vi "7_1_2.vi"() -> ()   [LabVIEW 2021, in "2022.lvlib"]
uses:
  2022.lvlib
  <vilib>/National Instruments/Tree Map/Tree Map Data.ctl
  <vilib>/National Instruments/Tree Map/Tree Map.lvlib
panel:
  out "min value":i32
  out "Array 4":i32[](array[numeric])
  out "Array 3":string[](array[string])
  out "x = y? 2":bool
  out "x-y":i32
  out "sum":i32
  out "Array 2":i32[](array[numeric])
  out "Array":string[](array[string])
  out "x = y?":bool
  out "Tree Control Items":T1(array[cluster])
  out "size(s)":i32
  out "Numeric":i32
  out "Tree Map Out":T2
  in  "Tree Control":string(tree)
  out "substring":string
  out "subarray":string[](array[string])
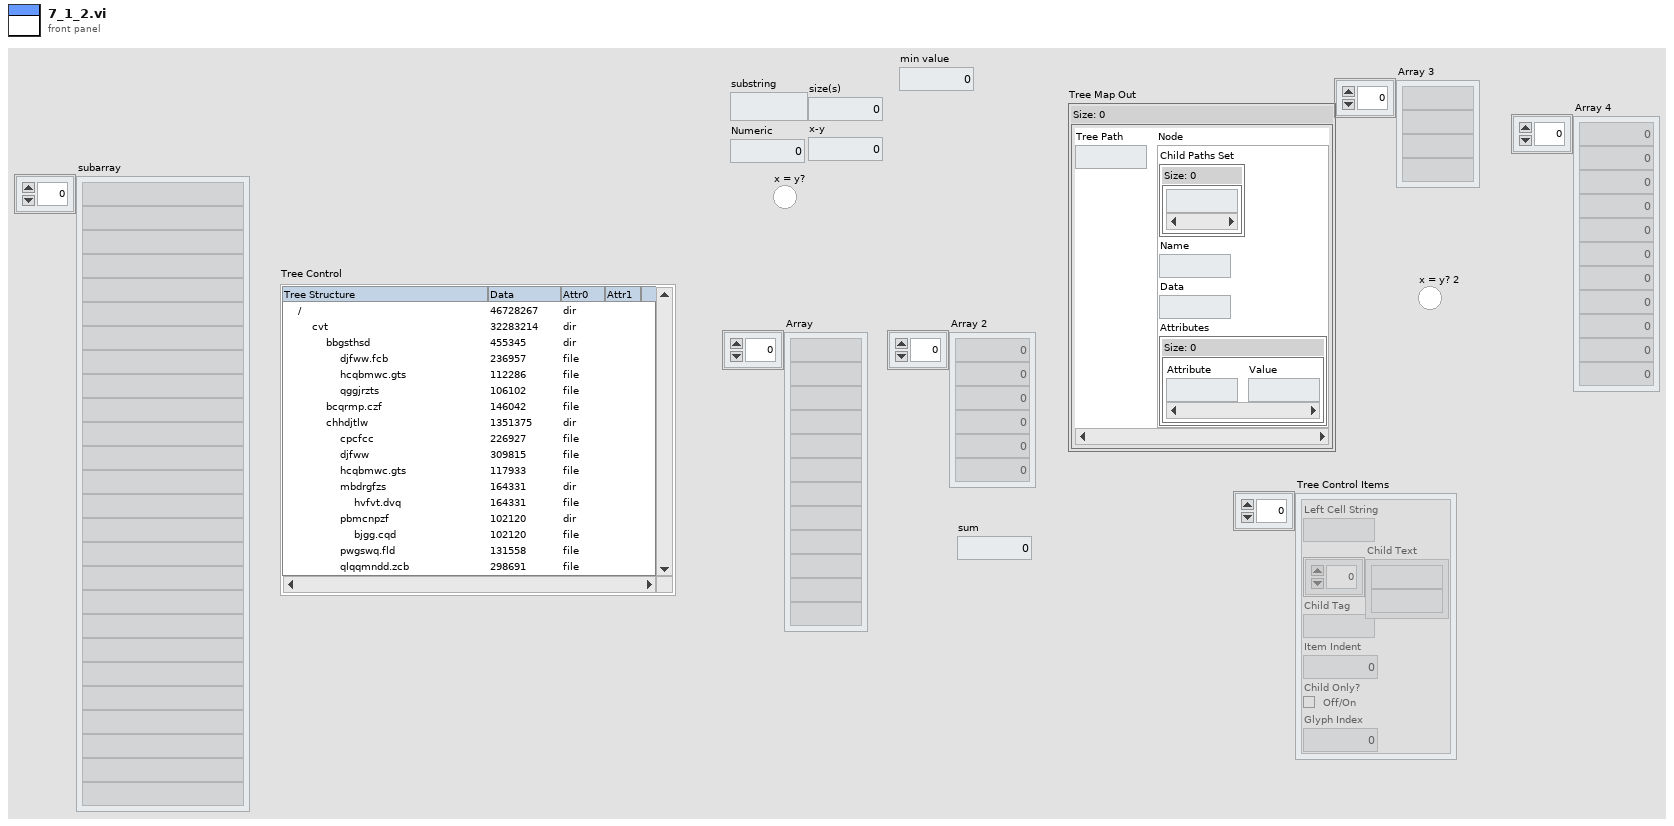
[diagram p1: front panel]
types:
  T1 = cluster{"Left Cell String":string, "Child Text":string[], "Child Tag":string, "Item Indent":i32, "Child Only?":bool, "Glyph Index":i32}[]
  T2 = typedef "Tree Map.lvlib/Tree Map Data.ctl" = map{string, cluster{"Child Paths Set":set{string}, "Name":string, "Data":string, "Attributes":map{string, string}}}
  T3 = cluster{"Child Paths Set":set{string}, "Name":string, "Data":string, "Attributes":map{string, string}}
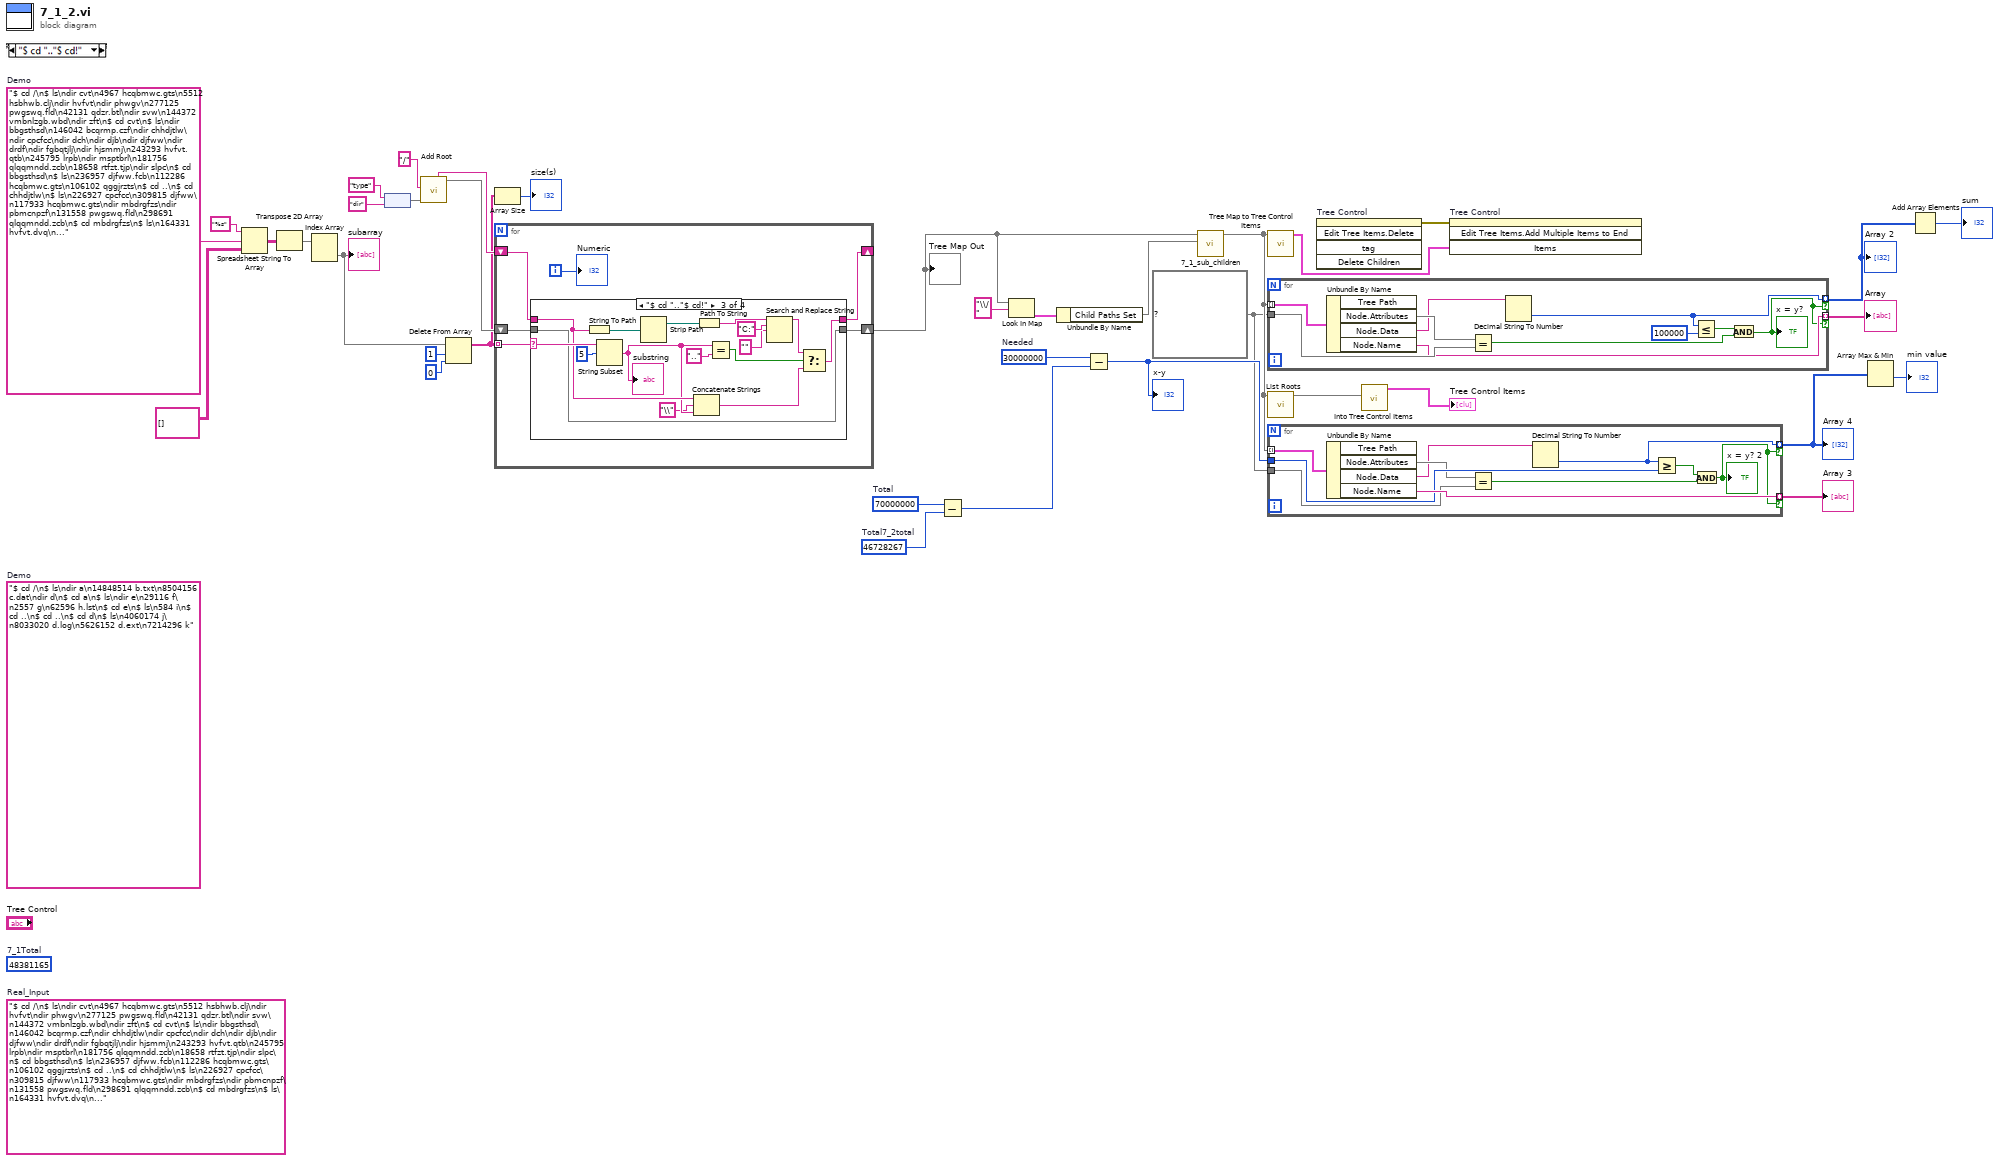
[diagram p0: block diagram]
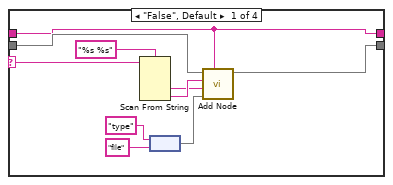
[diagram p2: hidden frame]
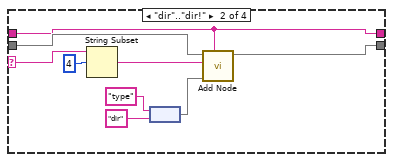
[diagram p3: hidden frame]
diagram:
  (unwired) 48381165  # 7_1Total
  w9 = 70000000  # Total
  w11 = 30000000  # Needed
  w1 = 46728267  # Total7_2total
  w2 = "$ cd /\n$ ls\ndir cvt\n4967 hcqbmwc.gts\n5512 hsbhwb.clj\ndir hvfvt\ndir phwgv\n277125 pwgswq.fld\n42131 qdzr.btl\ndir svw\n144372 vmbnlzgb.wbd\ndir zft\n$ cd cvt\n$ ls\ndir bbgsthsd\n146042 bcqrmp.czf\ndir chhdjtlw\ndir cpcfcc\ndir dch\ndir djb\ndir djfww\ndir drdf\ndir fgbqtjlj\ndir hjsmmj\n243293 hvfvt.qtb\n245795 lrpb\ndir msptbrl\n181756 qlqqmndd.zcb\n18658 rtfzt.tjp\ndir slpc\n$ cd bbgsthsd\n$ ls\n236957 djfww.fcb\n112286 hcqbmwc.gts\n106102 qggjrzts\n$ cd ..\n$ cd chhdjtlw\n$ ls\n226927 cpcfcc\n309815 djfww\n117933 hcqbmwc.gts\ndir mbdrgfzs\ndir pbmcnpzf\n131558 pwgswq.fld\n298691 qlqqmndd.zcb\n$ cd mbdrgfzs\n$ ls\n164331 hvfvt.dvq\n$ cd ..\n$ cd pbmcnpzf\n$ ls\n102120 bjgg.cqd\n$ cd ..\n$ cd ..\n$ cd cpcfcc\n$ ls\n15756 ddc\ndir dqc\ndir glm\ndir jbszm\n200345 pwgswq.fld\n145508 qlqqmndd.zcb\ndir vcptbw\ndir zrtm\n$ cd dqc\n$ ls\ndir cpcfcc\n92063 mzp\ndir qmhnvmh\ndir snqqcjlw\n8423 zdjwr.blc\n$ cd cpcfcc\n$ ls\ndir hvfvt\n$ cd hvfvt\n$ ls\n289372 pwgswq.fld\n307397 qlqqmndd.zcb\n$ cd ..\n$ cd ..\n$ cd qmhnvmh\n$ ls\n274778 jczjwdl.smd\n194322 ngrrfm\n$ cd ..\n$ cd snqqcjlw\n$ ls\n182851 nprvrgd.tbb\n$ cd ..\n$ cd ..\n$ cd glm\n$ ls\n188702 hpq.hgm\n$ cd ..\n$ cd jbszm\n$ ls\n187645 pwgswq.fld\n$ cd ..\n$ cd vcptbw\n$ ls\ndir mgqd\n$ cd mgqd\n$ ls\n157695 rhldvntj.jzm\n268696 rjnngctw\n$ cd ..\n$ cd ..\n$ cd zrtm\n$ ls\n218820 bcqrmp.czf\n172319 czpsl.dnf\n180114 hcqbmwc.gts\n165216 hvfvt.nnw\ndir zft\n$ cd zft\n$ ls\n161245 dtqjg.czv\n249888 hpq.hgm\n192037 zft\n$ cd ..\n$ cd ..\n$ cd ..\n$ cd dch\n$ ls\ndir djfww\ndir fzqgwwnf\ndir hqvmq\ndir mmcrzqc\n42136 qlqqmndd.zcb\ndir vdtlh\ndir wfltm\n271200 zrtm\n$ cd djfww\n$ ls\n37427 dct\n204401 hcqbmwc.gts\n283140 jmq\ndir lbrhbc\n154148 pncb.bmp\n53366 vzt.cnn\n$ cd lbrhbc\n$ ls\ndir djfww\n153648 djfww.pps\n308911 mvtjzp.btg\n219150 ncmc\n253604 wqft.ggb\n293759 zft\n$ cd djfww\n$ ls\n24794 hcqbmwc.gts\n$ cd ..\n$ cd ..\n$ cd ..\n$ cd fzqgwwnf\n$ ls\n233720 scdd.pwr\n$ cd ..\n$ cd hqvmq\n$ ls\ndir cdld\ndir cpcfcc\ndir djfww\n85564 hpq.hgm\ndir qnc\n81509 wtnl.crs\n$ cd cdld\n$ ls\n293421 llpltsgn.tqb\n$ cd ..\n$ cd cpcfcc\n$ ls\n230813 cglljgv\n178203 qlqqmndd.zcb\n186410 zrtm.tbt\n$ cd ..\n$ cd djfww\n$ ls\n201830 zrtm\n$ cd ..\n$ cd qnc\n$ ls\n305356 bdf.jrh\ndir zrtm\n$ cd zrtm\n$ ls\ndir bdhdrr\n$ cd bdhdrr\n$ ls\ndir nffdrnb\n$ cd nffdrnb\n$ ls\n301601 nbrjz\n$ cd ..\n$ cd ..\n$ cd ..\n$ cd ..\n$ cd ..\n$ cd mmcrzqc\n$ ls\ndir cpcfcc\n264271 hpq.hgm\n208744 tzsjrf.zdc\n274096 zft\n$ cd cpcfcc\n$ ls\n226054 cpcfcc\n$ cd ..\n$ cd ..\n$ cd vdtlh\n$ ls\n84229 bzlg.crn\n58668 cpcfcc.zqw\n141409 hpq.hgm\ndir mdgst\n37090 pstsh.qwv\n40357 qlqqmndd.zcb\ndir smr\ndir sqbgcsgh\ndir trp\n$ cd mdgst\n$ ls\n151033 fsmvbpsl.nqr\n$ cd ..\n$ cd smr\n$ ls\n140764 cpcfcc.dpg\n$ cd ..\n$ cd sqbgcsgh\n$ ls\ndir djfww\n263783 dvm\n105219 hpq.hgm\n29647 hwcgv.gvg\n162537 lwjhgh.wmt\n235511 nlw\ndir zwddrdfz\n$ cd djfww\n$ ls\n260084 vcgpvpd\n$ cd ..\n$ cd zwddrdfz\n$ ls\n225632 bhrzzw\n269756 cqq.vrz\n$ cd ..\n$ cd ..\n$ cd trp\n$ ls\n233192 vqwngcs\n$ cd ..\n$ cd ..\n$ cd wfltm\n$ ls\n140990 djfww\n$ cd ..\n$ cd ..\n$ cd djb\n$ ls\n213191 cjwrs.prd\ndir dhvpqt\ndir gtgftm\ndir hvfvt\n208325 jwhp\n301446 qlqqmndd.zcb\ndir qnlbgvf\ndir tps\ndir zft\ndir zrtm\ndir zwnlm\n$ cd dhvpqt\n$ ls\ndir sbcj\n$ cd sbcj\n$ ls\n20611 ggt\n$ cd ..\n$ cd ..\n$ cd gtgftm\n$ ls\n179526 qcqbtmvq\n$ cd ..\n$ cd hvfvt\n$ ls\ndir djstcnrt\ndir hggpvn\ndir hvfvt\n63889 hvfvt.tjm\n265836 qlqqmndd.zcb\n105663 zft\n223582 zft.llg\n26037 zzwwg.lqh\n$ cd djstcnrt\n$ ls\n201498 hcqbmwc.gts\n139156 hpq.hgm\n277342 pshgz.rtp\ndir rjb\n257294 rqrb.lhh\ndir tqnbfnt\n313308 zft.dvc\n$ cd rjb\n$ ls\n268438 hpq.hgm\ndir hvfvt\ndir hvwpb\n161024 mzbcgqc.nvw\n137875 pwgswq.fld\n260008 pzzcww\n283261 wnvlrg.tmn\n$ cd hvfvt\n$ ls\ndir dvwqqt\n163397 hcqbmwc.gts\n265154 pwgswq.fld\ndir trsh\ndir vnf\n$ cd dvwqqt\n$ ls\n315187 hcqbmwc.gts\n$ cd ..\n$ cd trsh\n$ ls\ndir ssrdpg\n$ cd ssrdpg\n$ ls\ndir vjdc\n$ cd vjdc\n$ ls\ndir srvdrhdq\n$ cd srvdrhdq\n$ ls\n74145 djfww\n$ cd ..\n$ cd ..\n$ cd ..\n$ cd ..\n$ cd vnf\n$ ls\ndir djfww\n$ cd djfww\n$ ls\n184018 pwgswq.fld\n$ cd ..\n$ cd ..\n$ cd ..\n$ cd hvwpb\n$ ls\ndir jwpjrcvs\n$ cd jwpjrcvs\n$ ls\ndir cpcfcc\n$ cd cpcfcc\n$ ls\n52191 sdlv\n$ cd ..\n$ cd ..\n$ cd ..\n$ cd ..\n$ cd tqnbfnt\n$ ls\ndir djfww\n206341 fmpb.lnp\ndir fpsjg\n4589 hcqbmwc.gts\ndir hvfvt\n8796 hvfvt.hdz\n238364 tgcdpjc.fjm\ndir zrtm\n40577 zrtm.fsr\n$ cd djfww\n$ ls\n217182 djfww.rbf\n$ cd ..\n$ cd fpsjg\n$ ls\n52456 djfww\n$ cd ..\n$ cd hvfvt\n$ ls\ndir rqhzvb\n275026 szwgzm.qjd\ndir zbmtstj\n$ cd rqhzvb\n$ ls\n8395 gcmzsd.jzf\n$ cd ..\n$ cd zbmtstj\n$ ls\n39691 qlqqmndd.zcb\ndir qqcdss\n180676 rwl.zwr\n$ cd qqcdss\n$ ls\n106297 zrtm.nsl\n$ cd ..\n$ cd ..\n$ cd ..\n$ cd zrtm\n$ ls\n153478 ldhvt\n$ cd ..\n$ cd ..\n$ cd ..\n$ cd hggpvn\n$ ls\n19109 cpcfcc.fbh\n249168 fnqjc\n207420 qgzsh.pfs\n135472 qlqqmndd.zcb\n$ cd ..\n$ cd hvfvt\n$ ls\ndir djfww\n213659 hcqbmwc.gts\ndir jzdwq\n204021 nvbgf\n185328 qlqqmndd.zcb\ndir zrtm\n$ cd djfww\n$ ls\n180713 rwmm.gjt\n$ cd ..\n$ cd jzdwq\n$ ls\n57424 djfww.qtm\n104960 slq.bfp\n174906 svc\n$ cd ..\n$ cd zrtm\n$ ls\ndir mrtvhht\n$ cd mrtvhht\n$ ls\n188512 djfww.fvm\n$ cd ..\n$ cd ..\n$ cd ..\n$ cd ..\n$ cd qnlbgvf\n$ ls\ndir fjrhtssv\n46767 jhbnml.lpq\n$ cd fjrhtssv\n$ ls\n198664 fgcc\n245142 tsc.rsd\n$ cd ..\n$ cd ..\n$ cd tps\n$ ls\ndir fmlwghjv\n146731 gwch.ttr\ndir jjzmdd\ndir rtltrng\n191609 wff.mqt\n$ cd fmlwghjv\n$ ls\n189227 zrtm.vgg\n$ cd ..\n$ cd jjzmdd\n$ ls\ndir hvfvt\n178057 mpdfrrm\n49493 pwgswq.fld\n220129 sqgfb.flm\n231012 zrmsnmr\n$ cd hvfvt\n$ ls\ndir lbndbhc\n12602 mnclbss\n746 ppw\n$ cd lbndbhc\n$ ls\n49601 cdqvs.gwc\n158670 wvjpchjg\n$ cd ..\n$ cd ..\n$ cd ..\n$ cd rtltrng\n$ ls\ndir cpgh\n115613 hvfvt\n59441 zfs\n$ cd cpgh\n$ ls\ndir djfww\n$ cd djfww\n$ ls\ndir tgt\n$ cd tgt\n$ ls\ndir vqwvqss\n$ cd vqwvqss\n$ ls\ndir bsdrhz\n$ cd bsdrhz\n$ ls\ndir pld\n$ cd pld\n$ ls\n8543 mfs.gsb\n$ cd ..\n$ cd ..\n$ cd ..\n$ cd ..\n$ cd ..\n$ cd ..\n$ cd ..\n$ cd ..\n$ cd zft\n$ ls\ndir fhjgg\n$ cd fhjgg\n$ ls\n114494 pwgswq.fld\n$ cd ..\n$ cd ..\n$ cd zrtm\n$ ls\n201142 tlhr.rtd\n298232 wlcztszv\n$ cd ..\n$ cd zwnlm\n$ ls\n240023 hcqbmwc.gts\n159126 hpq.hgm\n22101 hvfvt.bfw\ndir ltzl\ndir mtfr\ndir sbw\ndir sqscdjlj\ndir ssf\n$ cd ltzl\n$ ls\n260692 hpq.hgm\n204540 hvfvt\n$ cd ..\n$ cd mtfr\n$ ls\n15391 pwgswq.fld\n$ cd ..\n$ cd sbw\n$ ls\n293226 hcqbmwc.gts\n267478 htllcq\n176349 nlbhcf.vpn\n286577 zft.gds\n$ cd ..\n$ cd sqscdjlj\n$ ls\n128776 gnh\ndir qbdpvcbt\n284505 qlsn.vdq\n$ cd qbdpvcbt\n$ ls\n280709 crv.hgm\n$ cd ..\n$ cd ..\n$ cd ssf\n$ ls\n13328 djfww.pjn\n19971 hvfvt\ndir zft\n$ cd zft\n$ ls\n97761 dnmnz\n$ cd ..\n$ cd ..\n$ cd ..\n$ cd ..\n$ cd djfww\n$ ls\n109590 bwfnnf.wpd\n297297 cmht.ljg\n280726 hvfvt\n$ cd ..\n$ cd drdf\n$ ls\n56764 pwgswq.fld\n300547 wqqm\n210698 zrtm.jvq\n$ cd ..\n$ cd fgbqtjlj\n$ ls\n22217 vrmgsz.ctg\n$ cd ..\n$ cd hjsmmj\n$ ls\n232911 bcqrmp.czf\n164656 hcqbmwc.gts\ndir jql\ndir ntd\ndir prgm\ndir psfvhh\ndir zft\n$ cd jql\n$ ls\n212767 zhnhn.lzm\ndir zrtm\n$ cd zrtm\n$ ls\n35950 bcqrmp.czf\n$ cd ..\n$ cd ..\n$ cd ntd\n$ ls\ndir vml\n$ cd vml\n$ ls\n60833 bcqrmp.czf\n$ cd ..\n$ cd ..\n$ cd prgm\n$ ls\n316166 pwgswq.fld\n$ cd ..\n$ cd psfvhh\n$ ls\n152195 pwgswq.fld\n92448 qlqqmndd.zcb\n$ cd ..\n$ cd zft\n$ ls\n95808 hpq.hgm\n$ cd ..\n$ cd ..\n$ cd msptbrl\n$ ls\n256069 hpq.hgm\n$ cd ..\n$ cd slpc\n$ ls\ndir djfww\n285380 djfww.gcm\n169898 hcqbmwc.gts\n40914 mnpnhpz\n188062 pwgswq.fld\ndir zrtm\n$ cd djfww\n$ ls\n94935 pwgswq.fld\n70655 qlqqmndd.zcb\n48528 zft.qvh\n$ cd ..\n$ cd zrtm\n$ ls\n160137 hcqbmwc.gts\n$ cd ..\n$ cd ..\n$ cd ..\n$ cd hvfvt\n$ ls\ndir cslthslv\n129407 prwq\ndir vrzfbtt\n$ cd cslthslv\n$ ls\ndir cpcfcc\n158361 hcqbmwc.gts\n$ cd cpcfcc\n$ ls\ndir zpgnczq\n$ cd zpgnczq\n$ ls\n158414 zft\n$ cd ..\n$ cd ..\n$ cd ..\n$ cd vrzfbtt\n$ ls\n185263 nqvvl\n$ cd ..\n$ cd ..\n$ cd phwgv\n$ ls\n253690 bzpcj.fcj\ndir wtbr\n168025 zdsh.tnq\n157840 zsdfqb.zbd\n$ cd wtbr\n$ ls\ndir lvgdb\n$ cd lvgdb\n$ ls\n177751 cpcfcc.dzr\n$ cd ..\n$ cd ..\n$ cd ..\n$ cd svw\n$ ls\ndir cpcfcc\n189430 hpq.hgm\ndir ntzbj\n13384 qlqqmndd.zcb\n10333 wdvqhwgl.trq\n161318 zwzp.jsn\n$ cd cpcfcc\n$ ls\n298999 hcqbmwc.gts\n290883 hpq.hgm\ndir qlnntp\ndir vpshs\n5547 wlrmg.bpc\ndir zft\n$ cd qlnntp\n$ ls\n168562 nqds.tqn\n$ cd ..\n$ cd vpshs\n$ ls\n246400 pwgswq.fld\n$ cd ..\n$ cd zft\n$ ls\n235634 hvfvt.hst\n$ cd ..\n$ cd ..\n$ cd ntzbj\n$ ls\n98777 qlqqmndd.zcb\n$ cd ..\n$ cd ..\n$ cd zft\n$ ls\ndir dhnzm\n299292 hvfvt.pvb\ndir ltfb\ndir mrvsjgsq\ndir ntr\ndir swmvhgd\ndir zrtm\n$ cd dhnzm\n$ ls\n267041 bbsj\n$ cd ..\n$ cd ltfb\n$ ls\n242136 bcqrmp.czf\n314862 dgdz\n203160 hcqbmwc.gts\n80422 hgvz\ndir qftjfqfv\n180815 sstl.wzg\ndir wmhm\ndir zft\ndir zszp\n$ cd qftjfqfv\n$ ls\ndir bmmw\n$ cd bmmw\n$ ls\ndir hvfvt\n318039 hvfvt.whc\n17057 pwgswq.fld\n$ cd hvfvt\n$ ls\n170348 brplf.wgv\n156783 hcqbmwc.gts\n$ cd ..\n$ cd ..\n$ cd ..\n$ cd wmhm\n$ ls\n178474 bcqrmp.czf\ndir cmsgv\ndir dcfvrtj\n225393 htjflrs.tlm\ndir hvfvt\ndir nlrs\n273173 nsmdd.glc\n151259 pwgswq.fld\ndir ztqvwjr\n$ cd cmsgv\n$ ls\ndir flgjbjg\n$ cd flgjbjg\n$ ls\n13971 cpcfcc\n20601 qlqqmndd.zcb\n$ cd ..\n$ cd ..\n$ cd dcfvrtj\n$ ls\n141992 djfww.djn\n118149 hpq.hgm\ndir qrmqslq\n$ cd qrmqslq\n$ ls\n105940 zrtm.vql\n$ cd ..\n$ cd ..\n$ cd hvfvt\n$ ls\n181962 hpq.hgm\n$ cd ..\n$ cd nlrs\n$ ls\n82705 vnfwjf.hhl\n$ cd ..\n$ cd ztqvwjr\n$ ls\n98257 pwgswq.fld\n83864 scv.pbp\n$ cd ..\n$ cd ..\n$ cd zft\n$ ls\n183072 rsbfsl.zsj\n$ cd ..\n$ cd zszp\n$ ls\ndir hvfvt\n$ cd hvfvt\n$ ls\ndir djfww\ndir dqdtgjtg\ndir hvfvt\n$ cd djfww\n$ ls\n117037 rnmbsq.zph\n259243 zrtm.znf\n$ cd ..\n$ cd dqdtgjtg\n$ ls\ndir lrbsvng\n59301 zft\n$ cd lrbsvng\n$ ls\n46301 bcqrmp.czf\n$ cd ..\n$ cd ..\n$ cd hvfvt\n$ ls\n223277 qlqqmndd.zcb\n$ cd ..\n$ cd ..\n$ cd ..\n$ cd ..\n$ cd mrvsjgsq\n$ ls\n160189 cpcfcc\ndir lzqf\n232626 pwgswq.fld\ndir rpmfcg\n$ cd lzqf\n$ ls\n135552 bcqrmp.czf\n48083 qlqqmndd.zcb\ndir rbg\n229086 rdswb.cjz\n204486 spbwfrwf.cmj\n$ cd rbg\n$ ls\ndir sjdwsbqq\n$ cd sjdwsbqq\n$ ls\n270621 rhv.shw\n$ cd ..\n$ cd ..\n$ cd ..\n$ cd rpmfcg\n$ ls\n227216 bld.jtn\ndir zft\n$ cd zft\n$ ls\n43056 vzc\n$ cd ..\n$ cd ..\n$ cd ..\n$ cd ntr\n$ ls\ndir cmtnqb\ndir djfww\n195371 wffvmql.lrv\n$ cd cmtnqb\n$ ls\n135380 pbng.vhq\n$ cd ..\n$ cd djfww\n$ ls\ndir fmvrrrq\ndir mbhrbss\ndir zrtm\n$ cd fmvrrrq\n$ ls\ndir cpcfcc\n79110 djfww\n300581 ftcdj.wcc\n$ cd cpcfcc\n$ ls\n234211 zsgsm\n$ cd ..\n$ cd ..\n$ cd mbhrbss\n$ ls\n149184 djfww.gwh\n185815 rhgw.rmj\n$ cd ..\n$ cd zrtm\n$ ls\ndir zft\n$ cd zft\n$ ls\n310043 bnwvt.fbg\n$ cd ..\n$ cd ..\n$ cd ..\n$ cd ..\n$ cd swmvhgd\n$ ls\n77547 djfww.jwr\n318547 drggg\n300962 pwgswq.fld\n$ cd ..\n$ cd zrtm\n$ ls\n229319 bflnffjj\ndir djfww\n142526 hvfvt\n232722 jprrf\n94024 ndmf.hdr\ndir vhdhn\n$ cd djfww\n$ ls\n30770 bcqrmp.czf\n$ cd ..\n$ cd vhdhn\n$ ls\ndir djfww\n48261 djfww.frg\ndir gqc\n316163 qlqqmndd.zcb\n$ cd djfww\n$ ls\n104095 cvjlthn.cfl\n223454 hgqwzh\n24715 pwgswq.fld\n283499 qlqqmndd.zcb\ndir zft\n224574 zlnwn\n$ cd zft\n$ ls\n100941 pwgswq.fld\n$ cd ..\n$ cd ..\n$ cd gqc\n$ ls\n156273 wpgwrdl"  # Demo
  w5 = map{string, string} {"type"="dir"} ("Attributes")
  (unwired) "$ cd /\n$ ls\ndir cvt\n4967 hcqbmwc.gts\n5512 hsbhwb.clj\ndir hvfvt\ndir phwgv\n277125 pwgswq.fld\n42131 qdzr.btl\ndir svw\n144372 vmbnlzgb.wbd\ndir zft\n$ cd cvt\n$ ls\ndir bbgsthsd\n146042 bcqrmp.czf\ndir chhdjtlw\ndir cpcfcc\ndir dch\ndir djb\ndir djfww\ndir drdf\ndir fgbqtjlj\ndir hjsmmj\n243293 hvfvt.qtb\n245795 lrpb\ndir msptbrl\n181756 qlqqmndd.zcb\n18658 rtfzt.tjp\ndir slpc\n$ cd bbgsthsd\n$ ls\n236957 djfww.fcb\n112286 hcqbmwc.gts\n106102 qggjrzts\n$ cd ..\n$ cd chhdjtlw\n$ ls\n226927 cpcfcc\n309815 djfww\n117933 hcqbmwc.gts\ndir mbdrgfzs\ndir pbmcnpzf\n131558 pwgswq.fld\n298691 qlqqmndd.zcb\n$ cd mbdrgfzs\n$ ls\n164331 hvfvt.dvq\n$ cd ..\n$ cd pbmcnpzf\n$ ls\n102120 bjgg.cqd\n$ cd ..\n$ cd ..\n$ cd cpcfcc\n$ ls\n15756 ddc\ndir dqc\ndir glm\ndir jbszm\n200345 pwgswq.fld\n145508 qlqqmndd.zcb\ndir vcptbw\ndir zrtm\n$ cd dqc\n$ ls\ndir cpcfcc\n92063 mzp\ndir qmhnvmh\ndir snqqcjlw\n8423 zdjwr.blc\n$ cd cpcfcc\n$ ls\ndir hvfvt\n$ cd hvfvt\n$ ls\n289372 pwgswq.fld\n307397 qlqqmndd.zcb\n$ cd ..\n$ cd ..\n$ cd qmhnvmh\n$ ls\n274778 jczjwdl.smd\n194322 ngrrfm\n$ cd ..\n$ cd snqqcjlw\n$ ls\n182851 nprvrgd.tbb\n$ cd ..\n$ cd ..\n$ cd glm\n$ ls\n188702 hpq.hgm\n$ cd ..\n$ cd jbszm\n$ ls\n187645 pwgswq.fld\n$ cd ..\n$ cd vcptbw\n$ ls\ndir mgqd\n$ cd mgqd\n$ ls\n157695 rhldvntj.jzm\n268696 rjnngctw\n$ cd ..\n$ cd ..\n$ cd zrtm\n$ ls\n218820 bcqrmp.czf\n172319 czpsl.dnf\n180114 hcqbmwc.gts\n165216 hvfvt.nnw\ndir zft\n$ cd zft\n$ ls\n161245 dtqjg.czv\n249888 hpq.hgm\n192037 zft\n$ cd ..\n$ cd ..\n$ cd ..\n$ cd dch\n$ ls\ndir djfww\ndir fzqgwwnf\ndir hqvmq\ndir mmcrzqc\n42136 qlqqmndd.zcb\ndir vdtlh\ndir wfltm\n271200 zrtm\n$ cd djfww\n$ ls\n37427 dct\n204401 hcqbmwc.gts\n283140 jmq\ndir lbrhbc\n154148 pncb.bmp\n53366 vzt.cnn\n$ cd lbrhbc\n$ ls\ndir djfww\n153648 djfww.pps\n308911 mvtjzp.btg\n219150 ncmc\n253604 wqft.ggb\n293759 zft\n$ cd djfww\n$ ls\n24794 hcqbmwc.gts\n$ cd ..\n$ cd ..\n$ cd ..\n$ cd fzqgwwnf\n$ ls\n233720 scdd.pwr\n$ cd ..\n$ cd hqvmq\n$ ls\ndir cdld\ndir cpcfcc\ndir djfww\n85564 hpq.hgm\ndir qnc\n81509 wtnl.crs\n$ cd cdld\n$ ls\n293421 llpltsgn.tqb\n$ cd ..\n$ cd cpcfcc\n$ ls\n230813 cglljgv\n178203 qlqqmndd.zcb\n186410 zrtm.tbt\n$ cd ..\n$ cd djfww\n$ ls\n201830 zrtm\n$ cd ..\n$ cd qnc\n$ ls\n305356 bdf.jrh\ndir zrtm\n$ cd zrtm\n$ ls\ndir bdhdrr\n$ cd bdhdrr\n$ ls\ndir nffdrnb\n$ cd nffdrnb\n$ ls\n301601 nbrjz\n$ cd ..\n$ cd ..\n$ cd ..\n$ cd ..\n$ cd ..\n$ cd mmcrzqc\n$ ls\ndir cpcfcc\n264271 hpq.hgm\n208744 tzsjrf.zdc\n274096 zft\n$ cd cpcfcc\n$ ls\n226054 cpcfcc\n$ cd ..\n$ cd ..\n$ cd vdtlh\n$ ls\n84229 bzlg.crn\n58668 cpcfcc.zqw\n141409 hpq.hgm\ndir mdgst\n37090 pstsh.qwv\n40357 qlqqmndd.zcb\ndir smr\ndir sqbgcsgh\ndir trp\n$ cd mdgst\n$ ls\n151033 fsmvbpsl.nqr\n$ cd ..\n$ cd smr\n$ ls\n140764 cpcfcc.dpg\n$ cd ..\n$ cd sqbgcsgh\n$ ls\ndir djfww\n263783 dvm\n105219 hpq.hgm\n29647 hwcgv.gvg\n162537 lwjhgh.wmt\n235511 nlw\ndir zwddrdfz\n$ cd djfww\n$ ls\n260084 vcgpvpd\n$ cd ..\n$ cd zwddrdfz\n$ ls\n225632 bhrzzw\n269756 cqq.vrz\n$ cd ..\n$ cd ..\n$ cd trp\n$ ls\n233192 vqwngcs\n$ cd ..\n$ cd ..\n$ cd wfltm\n$ ls\n140990 djfww\n$ cd ..\n$ cd ..\n$ cd djb\n$ ls\n213191 cjwrs.prd\ndir dhvpqt\ndir gtgftm\ndir hvfvt\n208325 jwhp\n301446 qlqqmndd.zcb\ndir qnlbgvf\ndir tps\ndir zft\ndir zrtm\ndir zwnlm\n$ cd dhvpqt\n$ ls\ndir sbcj\n$ cd sbcj\n$ ls\n20611 ggt\n$ cd ..\n$ cd ..\n$ cd gtgftm\n$ ls\n179526 qcqbtmvq\n$ cd ..\n$ cd hvfvt\n$ ls\ndir djstcnrt\ndir hggpvn\ndir hvfvt\n63889 hvfvt.tjm\n265836 qlqqmndd.zcb\n105663 zft\n223582 zft.llg\n26037 zzwwg.lqh\n$ cd djstcnrt\n$ ls\n201498 hcqbmwc.gts\n139156 hpq.hgm\n277342 pshgz.rtp\ndir rjb\n257294 rqrb.lhh\ndir tqnbfnt\n313308 zft.dvc\n$ cd rjb\n$ ls\n268438 hpq.hgm\ndir hvfvt\ndir hvwpb\n161024 mzbcgqc.nvw\n137875 pwgswq.fld\n260008 pzzcww\n283261 wnvlrg.tmn\n$ cd hvfvt\n$ ls\ndir dvwqqt\n163397 hcqbmwc.gts\n265154 pwgswq.fld\ndir trsh\ndir vnf\n$ cd dvwqqt\n$ ls\n315187 hcqbmwc.gts\n$ cd ..\n$ cd trsh\n$ ls\ndir ssrdpg\n$ cd ssrdpg\n$ ls\ndir vjdc\n$ cd vjdc\n$ ls\ndir srvdrhdq\n$ cd srvdrhdq\n$ ls\n74145 djfww\n$ cd ..\n$ cd ..\n$ cd ..\n$ cd ..\n$ cd vnf\n$ ls\ndir djfww\n$ cd djfww\n$ ls\n184018 pwgswq.fld\n$ cd ..\n$ cd ..\n$ cd ..\n$ cd hvwpb\n$ ls\ndir jwpjrcvs\n$ cd jwpjrcvs\n$ ls\ndir cpcfcc\n$ cd cpcfcc\n$ ls\n52191 sdlv\n$ cd ..\n$ cd ..\n$ cd ..\n$ cd ..\n$ cd tqnbfnt\n$ ls\ndir djfww\n206341 fmpb.lnp\ndir fpsjg\n4589 hcqbmwc.gts\ndir hvfvt\n8796 hvfvt.hdz\n238364 tgcdpjc.fjm\ndir zrtm\n40577 zrtm.fsr\n$ cd djfww\n$ ls\n217182 djfww.rbf\n$ cd ..\n$ cd fpsjg\n$ ls\n52456 djfww\n$ cd ..\n$ cd hvfvt\n$ ls\ndir rqhzvb\n275026 szwgzm.qjd\ndir zbmtstj\n$ cd rqhzvb\n$ ls\n8395 gcmzsd.jzf\n$ cd ..\n$ cd zbmtstj\n$ ls\n39691 qlqqmndd.zcb\ndir qqcdss\n180676 rwl.zwr\n$ cd qqcdss\n$ ls\n106297 zrtm.nsl\n$ cd ..\n$ cd ..\n$ cd ..\n$ cd zrtm\n$ ls\n153478 ldhvt\n$ cd ..\n$ cd ..\n$ cd ..\n$ cd hggpvn\n$ ls\n19109 cpcfcc.fbh\n249168 fnqjc\n207420 qgzsh.pfs\n135472 qlqqmndd.zcb\n$ cd ..\n$ cd hvfvt\n$ ls\ndir djfww\n213659 hcqbmwc.gts\ndir jzdwq\n204021 nvbgf\n185328 qlqqmndd.zcb\ndir zrtm\n$ cd djfww\n$ ls\n180713 rwmm.gjt\n$ cd ..\n$ cd jzdwq\n$ ls\n57424 djfww.qtm\n104960 slq.bfp\n174906 svc\n$ cd ..\n$ cd zrtm\n$ ls\ndir mrtvhht\n$ cd mrtvhht\n$ ls\n188512 djfww.fvm\n$ cd ..\n$ cd ..\n$ cd ..\n$ cd ..\n$ cd qnlbgvf\n$ ls\ndir fjrhtssv\n46767 jhbnml.lpq\n$ cd fjrhtssv\n$ ls\n198664 fgcc\n245142 tsc.rsd\n$ cd ..\n$ cd ..\n$ cd tps\n$ ls\ndir fmlwghjv\n146731 gwch.ttr\ndir jjzmdd\ndir rtltrng\n191609 wff.mqt\n$ cd fmlwghjv\n$ ls\n189227 zrtm.vgg\n$ cd ..\n$ cd jjzmdd\n$ ls\ndir hvfvt\n178057 mpdfrrm\n49493 pwgswq.fld\n220129 sqgfb.flm\n231012 zrmsnmr\n$ cd hvfvt\n$ ls\ndir lbndbhc\n12602 mnclbss\n746 ppw\n$ cd lbndbhc\n$ ls\n49601 cdqvs.gwc\n158670 wvjpchjg\n$ cd ..\n$ cd ..\n$ cd ..\n$ cd rtltrng\n$ ls\ndir cpgh\n115613 hvfvt\n59441 zfs\n$ cd cpgh\n$ ls\ndir djfww\n$ cd djfww\n$ ls\ndir tgt\n$ cd tgt\n$ ls\ndir vqwvqss\n$ cd vqwvqss\n$ ls\ndir bsdrhz\n$ cd bsdrhz\n$ ls\ndir pld\n$ cd pld\n$ ls\n8543 mfs.gsb\n$ cd ..\n$ cd ..\n$ cd ..\n$ cd ..\n$ cd ..\n$ cd ..\n$ cd ..\n$ cd ..\n$ cd zft\n$ ls\ndir fhjgg\n$ cd fhjgg\n$ ls\n114494 pwgswq.fld\n$ cd ..\n$ cd ..\n$ cd zrtm\n$ ls\n201142 tlhr.rtd\n298232 wlcztszv\n$ cd ..\n$ cd zwnlm\n$ ls\n240023 hcqbmwc.gts\n159126 hpq.hgm\n22101 hvfvt.bfw\ndir ltzl\ndir mtfr\ndir sbw\ndir sqscdjlj\ndir ssf\n$ cd ltzl\n$ ls\n260692 hpq.hgm\n204540 hvfvt\n$ cd ..\n$ cd mtfr\n$ ls\n15391 pwgswq.fld\n$ cd ..\n$ cd sbw\n$ ls\n293226 hcqbmwc.gts\n267478 htllcq\n176349 nlbhcf.vpn\n286577 zft.gds\n$ cd ..\n$ cd sqscdjlj\n$ ls\n128776 gnh\ndir qbdpvcbt\n284505 qlsn.vdq\n$ cd qbdpvcbt\n$ ls\n280709 crv.hgm\n$ cd ..\n$ cd ..\n$ cd ssf\n$ ls\n13328 djfww.pjn\n19971 hvfvt\ndir zft\n$ cd zft\n$ ls\n97761 dnmnz\n$ cd ..\n$ cd ..\n$ cd ..\n$ cd ..\n$ cd djfww\n$ ls\n109590 bwfnnf.wpd\n297297 cmht.ljg\n280726 hvfvt\n$ cd ..\n$ cd drdf\n$ ls\n56764 pwgswq.fld\n300547 wqqm\n210698 zrtm.jvq\n$ cd ..\n$ cd fgbqtjlj\n$ ls\n22217 vrmgsz.ctg\n$ cd ..\n$ cd hjsmmj\n$ ls\n232911 bcqrmp.czf\n164656 hcqbmwc.gts\ndir jql\ndir ntd\ndir prgm\ndir psfvhh\ndir zft\n$ cd jql\n$ ls\n212767 zhnhn.lzm\ndir zrtm\n$ cd zrtm\n$ ls\n35950 bcqrmp.czf\n$ cd ..\n$ cd ..\n$ cd ntd\n$ ls\ndir vml\n$ cd vml\n$ ls\n60833 bcqrmp.czf\n$ cd ..\n$ cd ..\n$ cd prgm\n$ ls\n316166 pwgswq.fld\n$ cd ..\n$ cd psfvhh\n$ ls\n152195 pwgswq.fld\n92448 qlqqmndd.zcb\n$ cd ..\n$ cd zft\n$ ls\n95808 hpq.hgm\n$ cd ..\n$ cd ..\n$ cd msptbrl\n$ ls\n256069 hpq.hgm\n$ cd ..\n$ cd slpc\n$ ls\ndir djfww\n285380 djfww.gcm\n169898 hcqbmwc.gts\n40914 mnpnhpz\n188062 pwgswq.fld\ndir zrtm\n$ cd djfww\n$ ls\n94935 pwgswq.fld\n70655 qlqqmndd.zcb\n48528 zft.qvh\n$ cd ..\n$ cd zrtm\n$ ls\n160137 hcqbmwc.gts\n$ cd ..\n$ cd ..\n$ cd ..\n$ cd hvfvt\n$ ls\ndir cslthslv\n129407 prwq\ndir vrzfbtt\n$ cd cslthslv\n$ ls\ndir cpcfcc\n158361 hcqbmwc.gts\n$ cd cpcfcc\n$ ls\ndir zpgnczq\n$ cd zpgnczq\n$ ls\n158414 zft\n$ cd ..\n$ cd ..\n$ cd ..\n$ cd vrzfbtt\n$ ls\n185263 nqvvl\n$ cd ..\n$ cd ..\n$ cd phwgv\n$ ls\n253690 bzpcj.fcj\ndir wtbr\n168025 zdsh.tnq\n157840 zsdfqb.zbd\n$ cd wtbr\n$ ls\ndir lvgdb\n$ cd lvgdb\n$ ls\n177751 cpcfcc.dzr\n$ cd ..\n$ cd ..\n$ cd ..\n$ cd svw\n$ ls\ndir cpcfcc\n189430 hpq.hgm\ndir ntzbj\n13384 qlqqmndd.zcb\n10333 wdvqhwgl.trq\n161318 zwzp.jsn\n$ cd cpcfcc\n$ ls\n298999 hcqbmwc.gts\n290883 hpq.hgm\ndir qlnntp\ndir vpshs\n5547 wlrmg.bpc\ndir zft\n$ cd qlnntp\n$ ls\n168562 nqds.tqn\n$ cd ..\n$ cd vpshs\n$ ls\n246400 pwgswq.fld\n$ cd ..\n$ cd zft\n$ ls\n235634 hvfvt.hst\n$ cd ..\n$ cd ..\n$ cd ntzbj\n$ ls\n98777 qlqqmndd.zcb\n$ cd ..\n$ cd ..\n$ cd zft\n$ ls\ndir dhnzm\n299292 hvfvt.pvb\ndir ltfb\ndir mrvsjgsq\ndir ntr\ndir swmvhgd\ndir zrtm\n$ cd dhnzm\n$ ls\n267041 bbsj\n$ cd ..\n$ cd ltfb\n$ ls\n242136 bcqrmp.czf\n314862 dgdz\n203160 hcqbmwc.gts\n80422 hgvz\ndir qftjfqfv\n180815 sstl.wzg\ndir wmhm\ndir zft\ndir zszp\n$ cd qftjfqfv\n$ ls\ndir bmmw\n$ cd bmmw\n$ ls\ndir hvfvt\n318039 hvfvt.whc\n17057 pwgswq.fld\n$ cd hvfvt\n$ ls\n170348 brplf.wgv\n156783 hcqbmwc.gts\n$ cd ..\n$ cd ..\n$ cd ..\n$ cd wmhm\n$ ls\n178474 bcqrmp.czf\ndir cmsgv\ndir dcfvrtj\n225393 htjflrs.tlm\ndir hvfvt\ndir nlrs\n273173 nsmdd.glc\n151259 pwgswq.fld\ndir ztqvwjr\n$ cd cmsgv\n$ ls\ndir flgjbjg\n$ cd flgjbjg\n$ ls\n13971 cpcfcc\n20601 qlqqmndd.zcb\n$ cd ..\n$ cd ..\n$ cd dcfvrtj\n$ ls\n141992 djfww.djn\n118149 hpq.hgm\ndir qrmqslq\n$ cd qrmqslq\n$ ls\n105940 zrtm.vql\n$ cd ..\n$ cd ..\n$ cd hvfvt\n$ ls\n181962 hpq.hgm\n$ cd ..\n$ cd nlrs\n$ ls\n82705 vnfwjf.hhl\n$ cd ..\n$ cd ztqvwjr\n$ ls\n98257 pwgswq.fld\n83864 scv.pbp\n$ cd ..\n$ cd ..\n$ cd zft\n$ ls\n183072 rsbfsl.zsj\n$ cd ..\n$ cd zszp\n$ ls\ndir hvfvt\n$ cd hvfvt\n$ ls\ndir djfww\ndir dqdtgjtg\ndir hvfvt\n$ cd djfww\n$ ls\n117037 rnmbsq.zph\n259243 zrtm.znf\n$ cd ..\n$ cd dqdtgjtg\n$ ls\ndir lrbsvng\n59301 zft\n$ cd lrbsvng\n$ ls\n46301 bcqrmp.czf\n$ cd ..\n$ cd ..\n$ cd hvfvt\n$ ls\n223277 qlqqmndd.zcb\n$ cd ..\n$ cd ..\n$ cd ..\n$ cd ..\n$ cd mrvsjgsq\n$ ls\n160189 cpcfcc\ndir lzqf\n232626 pwgswq.fld\ndir rpmfcg\n$ cd lzqf\n$ ls\n135552 bcqrmp.czf\n48083 qlqqmndd.zcb\ndir rbg\n229086 rdswb.cjz\n204486 spbwfrwf.cmj\n$ cd rbg\n$ ls\ndir sjdwsbqq\n$ cd sjdwsbqq\n$ ls\n270621 rhv.shw\n$ cd ..\n$ cd ..\n$ cd ..\n$ cd rpmfcg\n$ ls\n227216 bld.jtn\ndir zft\n$ cd zft\n$ ls\n43056 vzc\n$ cd ..\n$ cd ..\n$ cd ..\n$ cd ntr\n$ ls\ndir cmtnqb\ndir djfww\n195371 wffvmql.lrv\n$ cd cmtnqb\n$ ls\n135380 pbng.vhq\n$ cd ..\n$ cd djfww\n$ ls\ndir fmvrrrq\ndir mbhrbss\ndir zrtm\n$ cd fmvrrrq\n$ ls\ndir cpcfcc\n79110 djfww\n300581 ftcdj.wcc\n$ cd cpcfcc\n$ ls\n234211 zsgsm\n$ cd ..\n$ cd ..\n$ cd mbhrbss\n$ ls\n149184 djfww.gwh\n185815 rhgw.rmj\n$ cd ..\n$ cd zrtm\n$ ls\ndir zft\n$ cd zft\n$ ls\n310043 bnwvt.fbg\n$ cd ..\n$ cd ..\n$ cd ..\n$ cd ..\n$ cd swmvhgd\n$ ls\n77547 djfww.jwr\n318547 drggg\n300962 pwgswq.fld\n$ cd ..\n$ cd zrtm\n$ ls\n229319 bflnffjj\ndir djfww\n142526 hvfvt\n232722 jprrf\n94024 ndmf.hdr\ndir vhdhn\n$ cd djfww\n$ ls\n30770 bcqrmp.czf\n$ cd ..\n$ cd vhdhn\n$ ls\ndir djfww\n48261 djfww.frg\ndir gqc\n316163 qlqqmndd.zcb\n$ cd djfww\n$ ls\n104095 cvjlthn.cfl\n223454 hgqwzh\n24715 pwgswq.fld\n283499 qlqqmndd.zcb\ndir zft\n224574 zlnwn\n$ cd zft\n$ ls\n100941 pwgswq.fld\n$ cd ..\n$ cd ..\n$ cd gqc\n$ ls\n156273 wpgwrdl"  # Real_Input
  (unwired) "$ cd /\n$ ls\ndir a\n14848514 b.txt\n8504156 c.dat\ndir d\n$ cd a\n$ ls\ndir e\n29116 f\n2557 g\n62596 h.lst\n$ cd e\n$ ls\n584 i\n$ cd ..\n$ cd ..\n$ cd d\n$ ls\n4060174 j\n8033020 d.log\n5626152 d.ext\n7214296 k"  # Demo
  n1 = Spreadsheet String To Array(format string="%s", spreadsheet string=w2, array type (2D Dbl)=string[][] []) -> (array=w35:string[][])  [unwired: 1 in]
  n2 = Transpose 2D Array(2D array=w35) -> (transposed array=w34:string[][])
  n3 = Index Array(array=w34) -> (element=w33:string[])  [unwired: 2 in]
  "subarray" <- w33
  n4 = node("type" ("key"), "dir" ("key")) -> (w21:map{string, string})
  n5 = call <vilib>:"Add Root.vi"("Root Attributes"=w21, "New Root Name"="/") -> ("Tree Map Out"=w31:T2, "Root Path"=w30:string)  [unwired: 8 in]
  n6 = Delete From Array(array=w33, length=1, index=0) -> (array with subset deleted=w25:string[])  [unwired: 1 out]
  n7 = Array Size(array=w25) -> (size(s)=→"size(s)":i32)
  n8 = for {
    tunnel: w25 -> [w43] mode=indexing
    shift-right: [w40] -> w16
    shift-left: w31 -> [w42]
    shift-right: [w39] -> _
    shift-left: w30 -> [w41]
    i -> [w38]
    n9 = case shown="\"$ cd \"..\"$ cd!\"" w43 {
      selector: w43 -> [w48 w61 w78 _]
      tunnel: w42 -> [w53 w62 w75 w80]
      tunnel: w41 -> [w44 w54 w67 w79]
      tunnel: [w49 w55 w75 w80] -> w40
      tunnel: [w44 w54 w74 w79] -> w39
      frame "False", Default {
        n10 = Scan From String(format string="%s %s", input string=w48) -> (output 1=w45:string, output 2=w46:string)  [unwired: 4 in, 3 out]
        n11 = node("type" ("key"), "file" ("key")) -> (w50:map{string, string})
        n12 = call <vilib>:"Add Node.vi"("Parent Path"=w44, "Attributes"=w50, "Data"=w45, "New Node Name"=w46, "Tree Map In"=w53) -> ("Tree Map Out"=w49:T2)  [unwired: 4 in, 2 out]
      }
      frame "dir".."dir!" {
        n13 = String Subset(string=w61, offset (0)=4) -> (substring=w59:string)  [unwired: 1 in]
        n14 = node("type" ("key"), "dir" ("key")) -> (w56:map{string, string})
        n15 = call <vilib>:"Add Node.vi"("Parent Path"=w54, "Attributes"=w56, "New Node Name"=w59, "Tree Map In"=w62) -> ("Tree Map Out"=w55:T2)  [unwired: 5 in, 2 out]
      }
      frame "$ cd ".."$ cd!" {
        n16 = String To Path(string=w67) -> (path=w73:path)
        n17 = String Subset(string=w78, offset (0)=5) -> (substring=w66:string)  [unwired: 1 in]
        "substring" <- w66
        n18 = Strip Path(path=w73) -> (stripped path=w72:path)  [unwired: 1 out]
        n19 = Concatenate Strings(w67, "\\" ("string"), w66) -> (w65:string)
        n20 = Path To String(path=w72) -> (string=w71:string)
        n21 = Equal?(x=w66, y="..") -> (x = y?=w63:bool)
        n22 = Search and Replace String(input string=w71, search string="C:", replace string="" ("replace string (\"\")")) -> (result string=w69:string)  [unwired: 5 in, 3 out]
        n23 = Select(t=w69, s=w63, f=w65) -> (s? t:f=w74:string)
      }
      frame "$ ls" {
      }
    }
    "Numeric" <- w38
  }
  "Tree Map Out" <- w16
  n24 = Subtract(x=w9, y=w1) -> (x-y=w10:i32)
  n25 = Look In Map(map=w16, key="\\/" ("New Root Name")) -> (value=w19:T3)  [unwired: 1 in, 1 out]
  n26 = Unbundle By Name(w19) -> ("Child Paths Set"=w15:set{string})
  n27 = Subtract(x=w11, y=w10) -> (x-y=w7:i32)
  "x-y" <- w7
  n28 = call "7_1_sub_children.vi"("Child Paths Set 2"=w15, "Tree Map Out"=w16) -> ("Tree Map Out 2"=w8:T2)  [unwired: 7 in, 2 out]
  n29 = call <vilib>:"Tree Map to Tree Control Items.vi"("Tree Map In"=w8) -> ("Tree Control Items"=w28:T1)  [unwired: 10 in]
  n30 = for {
    tunnel: w8 -> [w90] mode=indexing
    tunnel: w5 -> [w88]
    tunnel: [w87] -> w14 mode=indexing if=w81
    tunnel: [w82] -> w13 mode=indexing if=w81
    n31 = Unbundle By Name(w90) -> ("Node.Attributes"=w89:map{string, string}, "Node.Data"=w85:string, "Node.Name"=w87:string)  [unwired: 1 out]
    n32 = Equal?(x=w89, y=w88) -> (x = y?=w86:bool)
    n33 = Decimal String To Number(string=w85) -> (number=w82:i32)  [unwired: 2 in, 1 out]
    n34 = Less Or Equal?(x=w82, y=100000) -> (x <= y?=w83:bool)
    n35 = And(x=w83, y=w86) -> (x .and. y?=w81:bool)
    "x = y?" <- w81
  }
  "Array" <- w14
  "Array 2" <- w13
  n36 = call <vilib>:"List Roots.vi"("Tree Map In"=w8) -> ("Unique Root Paths Set"=w18:set{string})  [unwired: 10 in]
  n37 = for {
    tunnel: [w100] -> w6 mode=indexing if=w96
    tunnel: [w97] -> w4 mode=indexing if=w96
    tunnel: w8 -> [w95] mode=indexing
    tunnel: w7 -> [w94]
    tunnel: w5 -> [w93]
    n38 = Unbundle By Name(w95) -> ("Node.Attributes"=w92:map{string, string}, "Node.Data"=w91:string, "Node.Name"=w100:string)  [unwired: 1 out]
    n39 = Equal?(x=w92, y=w93) -> (x = y?=w99:bool)
    n40 = Decimal String To Number(string=w91) -> (number=w97:i32)  [unwired: 2 in, 1 out]
    n41 = Greater Or Equal?(x=w97, y=w94) -> (x >= y?=w98:bool)
    n42 = And(x=w98, y=w99) -> (x .and. y?=w96:bool)
    "x = y? 2" <- w96
  }
  "Array 3" <- w6
  "Array 4" <- w4
  n43 = invoke on="Tree Control" class="Tree (strict)" method="Edit Tree Items.Delete"() -> (error out=w29:errorcluster)  [unwired: 5 in, 4 out]
  n44 = call <vilib>:"Into Tree Control Items.vi"("Paths Set"=w18) -> ("Tree Control Item"=→"Tree Control Items":T1)  [unwired: 10 in]
  n45 = invoke on="Tree Control" class="Tree (strict)" method="Edit Tree Items.Add Multiple Items to End"(error in=w29, "Items"=w28) -> ()  [unwired: 2 in, 4 out]
  n46 = Array Max & Min(array=w4) -> (min value=→"min value":i32)  [unwired: 3 out]
  n47 = Add Array Elements(numeric array=w13) -> (sum=→"sum":i32)
